vi "PH_Cam_BaseClass.Close Image.vi"(0 "i ref in":refnum<vi>, 5 "error in":errorcluster) -> (14 "i ref out":refnum<vi>, 19 "error out":errorcluster)   [LabVIEW 2014, in "PH_Cam_BaseClass.lvlib"]
doc: "This VI removes an image from the desk top."
uses:
  PH_Cam_BaseClass.lvlib
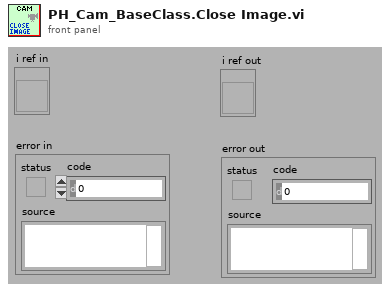
[diagram p1: front panel]
types:
  T1 = typedef "PH_Cam_BaseClass.lvlib/PH_Cam_BaseClass.i attribute.ctl" = cluster{"Gui Refs":T2, "Cam":cluster{"Source Notifier":refnum<notifier>, "Error":errorcluster, "Camera ID":string}, "Images":cluster{"Cam":T3, "Operation":T3, "PSDB":T3}, "Window Image":cluster{"Indicate Image":bool, "Window No.":i32, "Scale Facor":dbl, "Center Cross":bool, "Subtract Backgr":bool, "CoG":bool, "Color Palette":cluster{"Red":u8, "Green":u8, "Blue":u8}[], "Image On":bool}, "Default Prdc Int":i32, "Performance":cluster{"on":bool, "Timestamp Last Frame":i32}, "Histogram":cluster{"on":bool, "Mapping":bool}, "Save Image":cluster{"Save":bool, "File refnum":refnum<file>}, "Setting Service ID":i32, "Screen":cluster{"x-resolution":i16, "y-resolution":i16}, "On":bool, "Constructor finished":bool, "configured":bool}
  T2 = typedef "PH_Cam_BaseClass.lvlib/PH_Cam_BaseClass.GUI Refs.ctl" = cluster{"Frame Rate":refnum<vi>, "Get Frame Rate":refnum<vi>, "Show Image":refnum<vi>, "Get Histogram":refnum<vi>, "Mapping":refnum<vi>, "Histogram":refnum<vi>, "Center Cross":refnum<vi>, "Center of Gravity":refnum<vi>, "Scale Factor [%]":refnum<vi>, "Save Image":refnum<vi>, "Palette":refnum<vi>, "Subtract Background":refnum<vi>, "Cam Error":refnum<vi>, "On":refnum<vi>, "Cam List":refnum<vi>}
  T3 = typedef "IMAQ Image.ctl" = refnum<image>
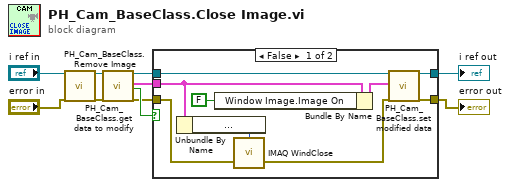
[diagram p0: block diagram]
diagram:
  n1 = call "PH_Cam_BaseClass.Remove Image.vi"("i ref in"="i ref in", "error in"="error in") -> ("i ref out"=w2:refnum<vi>, "error out"=w1:errorcluster)  [unwired: 16 in]
  n2 = call "PH_Cam_BaseClass.get data to modify.vi"("i ref in"=w2, "error in (no error)"=w1) -> ("i ref out"=w7:refnum<vi>, "i attribute"=w6:T1, "timed out"=w10:bool, "error out"=w5:errorcluster)  [unwired: 14 in]
  n3 = case shown="False" w10 {
    tunnel: w5 -> [w18 w20]
    tunnel: w6 -> [w13 _]
    tunnel: w7 -> [w17 w21]
    tunnel: [w16 w21] -> w8
    tunnel: [w14 w20] -> w9
    frame False {
      n4 = Unbundle By Name(w13) -> ("Window Image.Window No."=w19:i32)
      n5 = Bundle By Name(cluster=w13, "Window Image.Image On"=FALSE) -> (w12:T1)
      n6 = call "IMAQ WindClose"("Window Number (0...15)"=w19, "error in (no error)"=w18) -> ("error out"=w15:errorcluster)  [unwired: 4 in]
      n7 = call "PH_Cam_BaseClass.set modified data.vi"("i ref in"=w17, "i attribute"=w12, "error in (no error)"=w15) -> ("i ref out"=w16:refnum<vi>, "error out"=w14:errorcluster)  [unwired: 15 in]
    }
    frame True {
    }
  }
  "error out" <- w9
  "i ref out" <- w8
